vi "Monero-3.vi"() -> ()   [LabVIEW 2017, in "Monero-FPGA-3.lvlib"]
uses:
  Monero-FPGA-3.lvlib
  monero-3-control.ctl
  monero-3-data.ctl
  <vilib>/Platform/TimedLoop/XDataNode/timing_clust.ctl
  <vilib>/Platform/TimedLoop/XDataNode/nitl_modes.ctl
  <vilib>/Platform/TimedLoop/XDataNode/wakeup.ctl
  <vilib>/rvi/Emulation/niFpgaSctlEmulationGetInTimedLoop.vi
  <vilib>/rvi/Emulation/niFpgaEmulationReportErrorSimple.vi
  <vilib>/rvi/Emulation/niFpgaGetClockAttributes.vi
  <vilib>/rvi/Emulation/niFpgaCriticalErrorInLSC.vi
  <vilib>/rvi/interface/RandomDataEmulation/nirviRandomDataMultiElementFPGAFIFO.vi
  <instcachedir>/0/nirviRandomDataMultiElementFPGAFIFO_6740B454F3C245F78F76ED91F73FD8DB.lvgen/nirviRandomDataMultiElementFPGAFIFO_6740B454F3C245F78F76ED91F73FD8DB_003.vi
  <vilib>/rvi/interface/RandomDataEmulation/niFpgaRandomDataHandleErrors.vi
  <vilib>/Platform/TimedLoop/XDataNode/XDataNode.xnode
  <vilib>/rvi/DataTransferAndStorage/Container/XNode/niFpgaContainer.xnode
  <vilib>/rvi/interface/RandomDataEmulation/nirviRandomDataFpgaMultiElementTemplate.vi
  <vilib>/Platform/TimedLoop/XDataNode/XDNodeRunTimeDep.lvlib
panel:
  out "monero-3-data":T1
  out "monero-3-control":T2
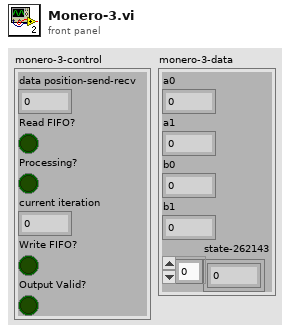
[diagram p1: front panel]
types:
  T1 = typedef "Monero-FPGA-3.lvlib/monero-3-data.ctl" = cluster{"a0":u64, "a1":u64, "b0":u64, "b1":u64, "state-262143":u64[]}
  T2 = typedef "Monero-FPGA-3.lvlib/monero-3-control.ctl" = cluster{"data position-send-recv":i32, "Read FIFO?":bool, "Processing?":bool, "current iteration":u32, "Write FIFO?":bool, "Output Valid?":bool}
  T3 = typedef "XDNodeRunTimeDep.lvlib/timing_clust.ctl" = cluster{"Expected End [f-1]":u64, "Actual End [f-1]":u64, "Finished Late? [f-1]":bool, "Expected End [i-1]":u64, "Actual End [i-1]":u64, "Finished Late? [i-1]":bool, "Expected Start [i]":u64, "Actual Start [i]":u64, "Expected Start [f]":u64, "Actual Start [f]":u64, "Source Name":string, "Structure Name":string, "Period":i64, "Deadline":i64, "Offset":i64, "Start":i64, "Priority":i32, "Timeout":i32, "Mode":T4, "Wakeup Reason":T5, "Error":errorcluster, "Source Type":string, "Secondary Source Type":string, "Global End Time":u64, "Global Start Time":u64, "Frame Duration":u64, "Iteration Duration":u64, "Assigned CPU":i32, "I/O Scan Engine Mode":u32}
  T4 = typedef "XDNodeRunTimeDep.lvlib/nitl_modes.ctl" = enum32{"No Change", "Process missed periods, maintain original phase", "Discard missed periods, maintain original phase", "Process missed periods, ignore original phase", "Discard missed periods, ignore original phase"}
  T5 = typedef "XDNodeRunTimeDep.lvlib/wakeup.ctl" = enum32{"Normal", "Aborted", "Asynchronous wakeup", "Timing source error", "Timed loop error", "Timeout"}
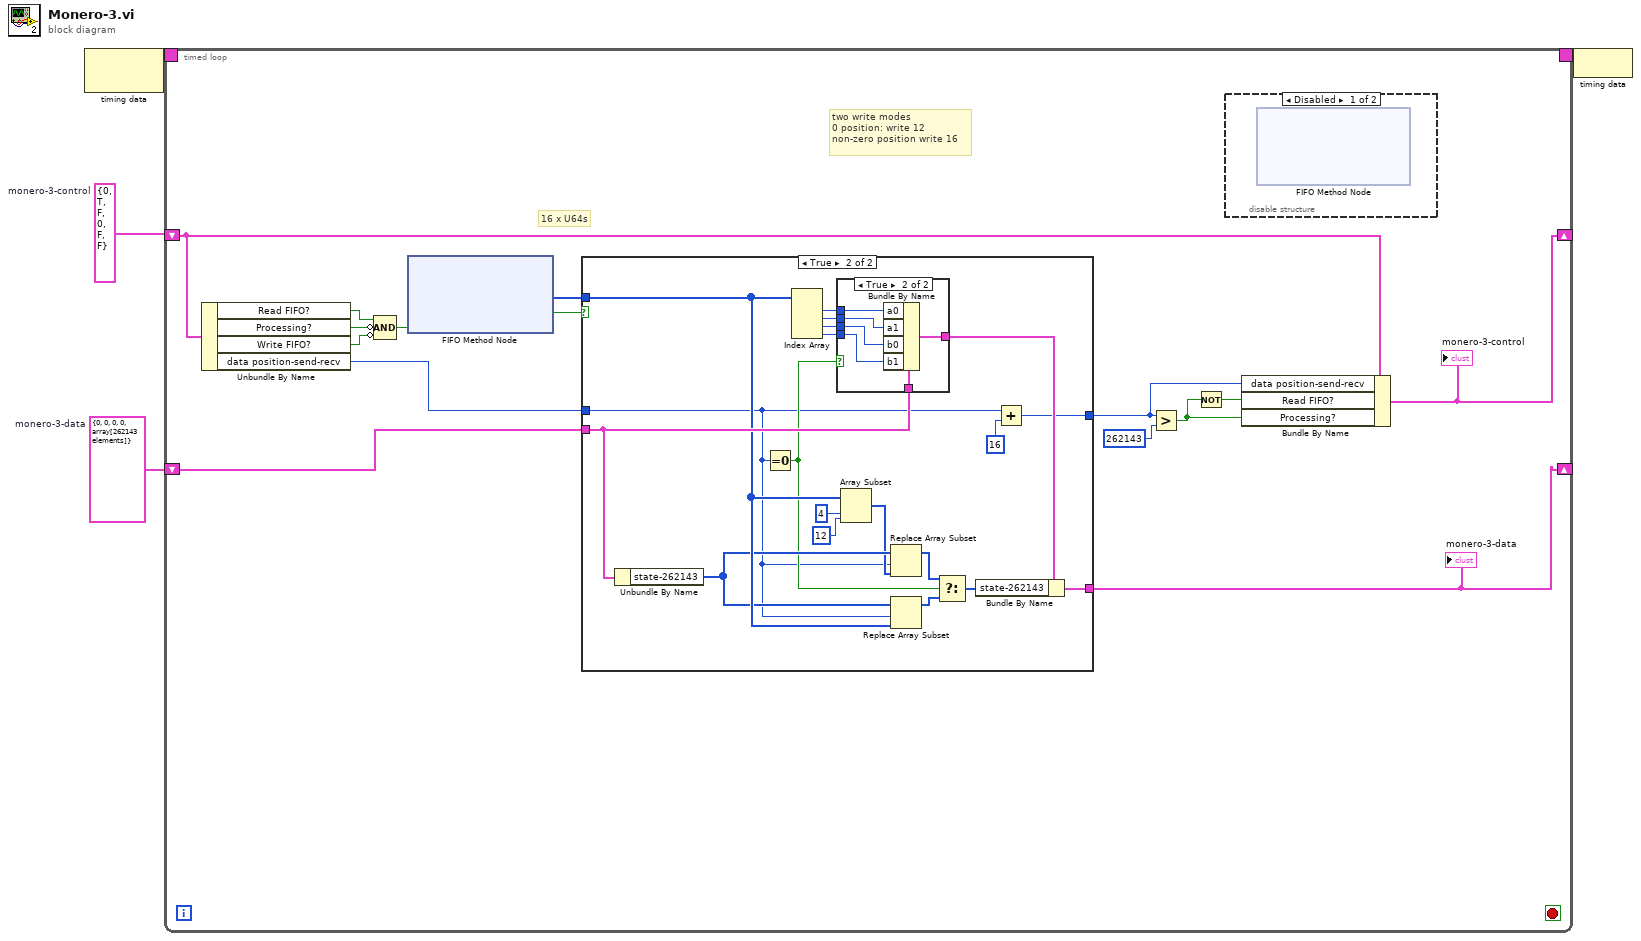
[diagram p0: block diagram]
diagram:
  w1 = T1 {"a0"=0, "a1"=0, "b0"=0, "b1"=0, "state-262143"=array[262143 elements]}  # monero-3-data
  w2 = T2 {"data position-send-recv"=0, "Read FIFO?"=TRUE, "Processing?"=FALSE, "current iteration"=0, "Write FIFO?"=FALSE, "Output Valid?"=FALSE}  # monero-3-control
  n1 = node-c288() -> (w4:T3)  [unwired: 1 in]
  n2 = timed-loop {
    timing: w4 -> [_]
    timing-out: [_] -> w3
    shift-right: [w6] -> _
    shift-left: w2 -> [w19]
    shift-right: [w5] -> _
    shift-left: w1 -> [w13]
    stop <- _ stop-if-true
    # "two write modes\n0 position: write 12\nnon-zero position write 16"
    # "16 x U64s"
    n3 = Unbundle By Name(w19) -> ("Read FIFO?"=w18:bool, "Processing?"=w17:bool, "Write FIFO?"=w16:bool, "data position-send-recv"=w11:i32)
    n4 = Compound Arithmetic op=AND(w18, invert w17, invert w16) -> (w15:bool)
    n5 = xnode ("FIFO Method Node")("Ready for Output"=w15) -> ("Element"=w12:u64[], "Output Valid"=w14:bool)  [unwired: 1 in, 1 out]
    n6 = case shown="True" w14 {
      tunnel: w13 -> [w21 w39]
      tunnel: [w21 w40] -> w5
      tunnel: w12 -> [_ w31]
      tunnel: w11 -> [w20 w22]
      tunnel: [w20 w23] -> w10
      frame False {
      }
      frame True {
        n7 = Unbundle By Name(w39) -> ("state-262143"=w30:u64[])
        n8 = Equal To 0?(x=w22) -> (x = 0?=w28:bool)
        n9 = Index Array(array=w31) -> (element #1=w37:u64, element #2=w36:u64, element #3=w35:u64, element #4=w34:u64)  [unwired: 4 in]
        n10 = case shown="True" w28 {
          tunnel: w39 -> [w41 w47]
          tunnel: [w41 w46] -> w38
          tunnel: w37 -> [_ w45]
          tunnel: w36 -> [_ w44]
          tunnel: w35 -> [_ w43]
          tunnel: w34 -> [_ w42]
          frame False {
          }
          frame True {
            n11 = Bundle By Name(cluster=w47, "a0"=w45, "a1"=w44, "b0"=w43, "b1"=w42) -> (w46:T1)
          }
        }
        n12 = Array Subset(array=w31, index=4, length=12) -> (w25:u64[])
        n13 = Replace Array Subset(array=w30, new element=w25, index=w22) -> (w27:u64[])
        n14 = Replace Array Subset(array=w30, new element=w31, index=w22) -> (w26:u64[])
        n15 = Select(t=w27, s=w28, f=w26) -> (s? t:f=w29:u64[])
        n16 = Bundle By Name(cluster=w38, "state-262143"=w29) -> (w40:T1)
        n17 = Add(x=w22, y=16) -> (x+y=w23:i32)
      }
    }
    "monero-3-data" <- w5
    n18 = Greater?(x=w10, y=262143 ("data position-send-recv")) -> (0:w9:bool)
    n19 = Not(x=w9) -> (.not. x?=w8:bool)
    n20 = disable-structure shown="Disabled" {
      frame Disabled {
        n21 = xnode ("FIFO Method Node")() -> ()  [unwired: 3 in, 2 out]
      }
      frame Enabled {
      }
    }
    n22 = Bundle By Name(cluster=w19, "data position-send-recv"=w10, "Read FIFO?"=w8, "Processing?"=w9) -> (w6:T2)
    "monero-3-control" <- w6
  }
  n23 = node-c288(w3) -> ()
